vi "Parse Log Entries.vi"(8 "error in (no error)":errorcluster, 11 "Split String":string[][](array[string])) -> (0 "error out":errorcluster, 3 "Day 4 Data":T1)   [LabVIEW 2019]
uses:
  Log Entry.ctl
  <vilib>/Utility/error.llb/Error Cluster From Error Code.vi
  <vilib>/regexp/Match Regular Expression.xnode
  <vilib>/ErrorRing/Error Ring.xnode
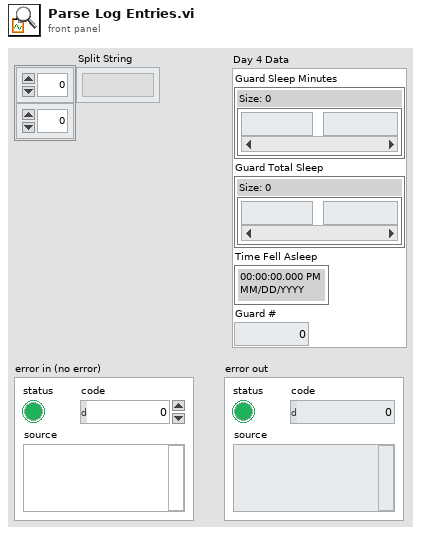
[diagram p1: front panel]
types:
  T1 = typedef "Log Entry.ctl" = cluster{"Guard Sleep Minutes":map{string, i32}, "Guard Total Sleep":map{string, i32}, "Time Fell Asleep":timestamp, "Guard #":i32}
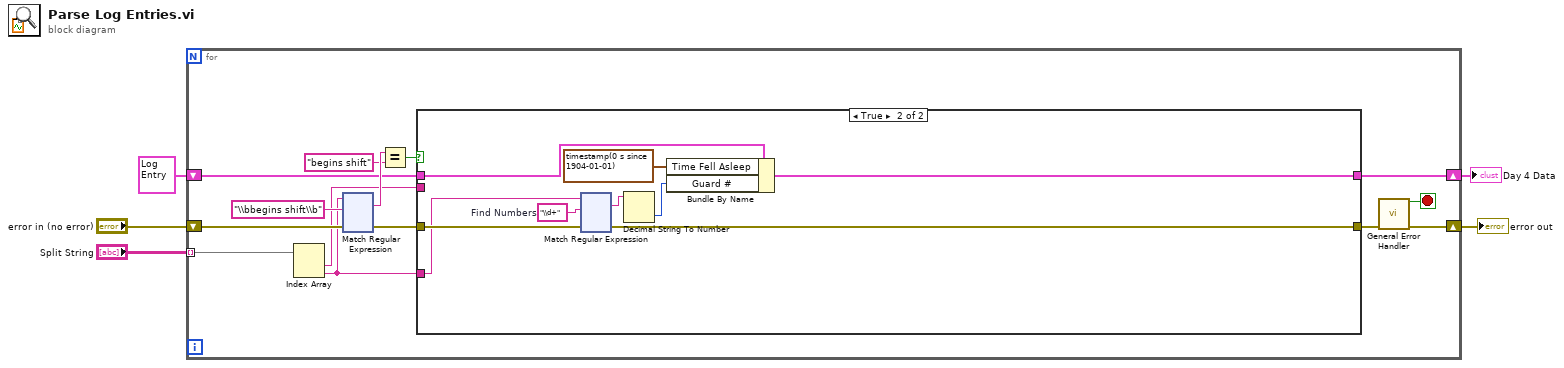
[diagram p0: block diagram]
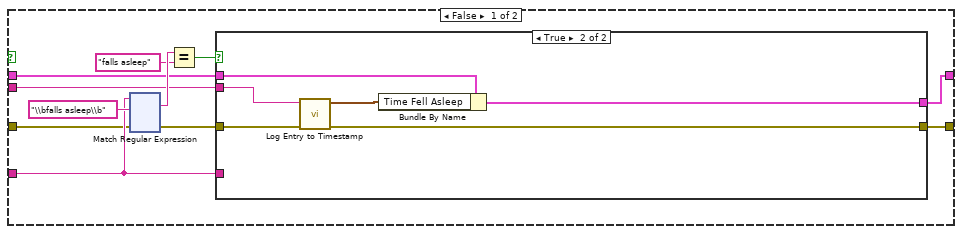
[diagram p2: hidden frame]
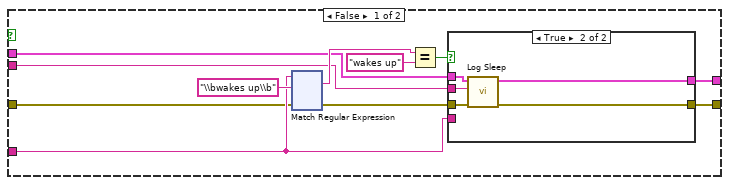
[diagram p3: hidden frame]
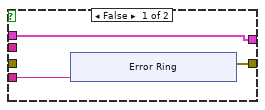
[diagram p4: hidden frame]
diagram:
  n1 = for {
    tunnel: "Split String" -> [w19] mode=indexing
    shift-right: [w10] -> w4
    shift-left: "error in (no error)" -> [w14]
    shift-right: [w6] -> w1
    shift-left: T1 {"Guard Sleep Minutes"={}, "Guard Total Sleep"={}, "Time Fell Asleep"=timestamp(0 s since 1904-01-01), "Guard #"=0} -> [w7]
    stop <- w8 stop-if-true
    n2 = Index Array(array=w19) -> (element #1=w11:string, element #2=w12:string)  [unwired: 2 in]
    n3 = xnode "Match Regular Expression"("input string"=w12, "regular expression"="\\bbegins shift\\b", "error in"=w14) -> ("whole match"=w17:string, "error out"=w13:errorcluster)  [unwired: 3 in, 3 out]
    n4 = Equal?(x=w17, y="begins shift") -> (x = y?=w15:bool)
    n5 = case shown="True" w15 {
      tunnel: w12 -> [w27 w297]
      tunnel: w13 -> [w25 w298]
      tunnel: [w22 w295] -> w9
      tunnel: w11 -> [w23 _]
      tunnel: w7 -> [w21 w294]
      tunnel: [w20 w291] -> w6
      frame False {
        n6 = xnode "Match Regular Expression"("input string"=w27, "regular expression"="\\bfalls asleep\\b", "error in"=w25) -> ("whole match"=w29:string, "error out"=w24:errorcluster)  [unwired: 3 in, 3 out]
        n7 = Equal?(x=w29, y="falls asleep") -> (x = y?=w26:bool)
        n8 = case shown="True" w26 {
          tunnel: w27 -> [w37 _]
          tunnel: w24 -> [w36 w175]
          tunnel: [w34 w174] -> w22
          tunnel: w23 -> [w33 w176]
          tunnel: w21 -> [w32 w173]
          tunnel: [w31 w171] -> w20
          frame False {
            n9 = xnode "Match Regular Expression"("input string"=w37, "regular expression"="\\bwakes up\\b", "error in"=w36) -> ("whole match"=w40:string, "error out"=w35:errorcluster)  [unwired: 3 in, 3 out]
            n10 = Equal?(x=w40, y="wakes up") -> (x = y?=w38:bool)
            n11 = case shown="True" w38 {
              tunnel: w37 -> [w44 _]
              tunnel: w35 -> [_ w56]
              tunnel: [w43 w54] -> w34
              tunnel: w33 -> [_ w55]
              tunnel: w32 -> [w42 w52]
              tunnel: [w42 w53] -> w31
              frame False {
                n12 = xnode "Error Ring"("parameter 0"=w44) -> ("error out"=w43:errorcluster)
              }
              frame True {
                n13 = call "Log Sleep.vi"("error in (no error)"=w56, "String"=w55, "Cluster in"=w52) -> ("error out"=w54:errorcluster, "Cluster out"=w53:T1)  [unwired: 7 in]
              }
            }
          }
          frame True {
            n14 = call "Log Entry to Timestamp.vi"("error in (no error)"=w175, "String"=w176) -> ("error out"=w174:errorcluster, "Time Stamp"=w172:timestamp)  [unwired: 8 in]
            n15 = Bundle By Name(cluster=w173, "Time Fell Asleep"=w172) -> (w171:T1)
          }
        }
      }
      frame True {
        w299 = "\\d+"  # Find Numbers
        n16 = xnode "Match Regular Expression"("input string"=w297, "regular expression"=w299, "error in"=w298) -> ("whole match"=w296:string, "error out"=w295:errorcluster)  [unwired: 3 in, 3 out]
        n17 = Decimal String To Number(string=w296) -> (number=w293:i32)  [unwired: 2 in, 1 out]
        n18 = Bundle By Name(cluster=w294, "Time Fell Asleep"=timestamp(0 s since 1904-01-01) ("Time Stamp"), "Guard #"=w293) -> (w291:T1)
      }
    }
    n19 = call <vilib>:"General Error Handler.vi"("error in (no error)"=w9) -> ("error?"=w8:bool, "error out"=w10:errorcluster)  [unwired: 10 in, 3 out]
  }
  "error out" <- w4
  "Day 4 Data" <- w1
